vi "menu-SetWeights.vi"(10 "Start":i32, 11 "Array in":T1[](array[typedef])) -> (3 "Array out":T1[](array[typedef]))   [LabVIEW 2019]
uses:
  <resource>/Framework/Providers/API/mxLvMenuItem.ctl
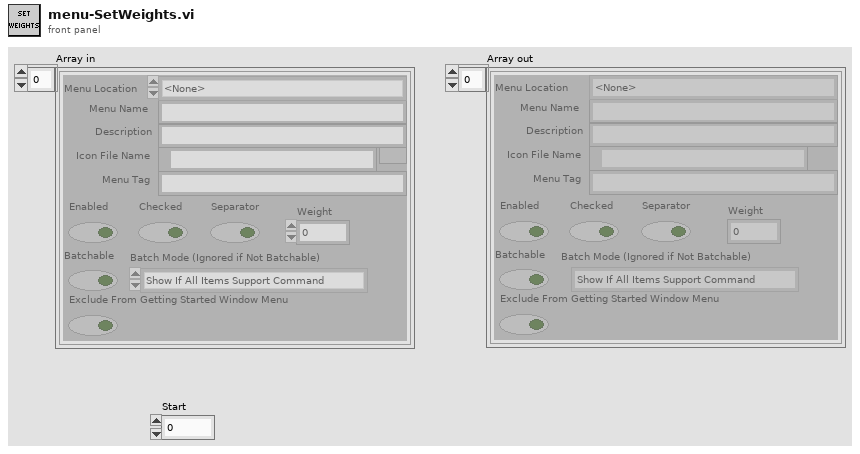
[diagram p1: front panel]
types:
  T1 = typedef "mxLvMenuItem.ctl" = cluster{"Menu Name":string, "Description":string, "Icon File Name":path, "Menu Tag":string, "Enabled":bool, "Checked":bool, "Separator":bool, "Batchable":bool, "Weight":i32, "Batch Mode (Ignored if Not Batchable)":enum32{"Show If All Items Support Command", "Show If Any Items Support Command"}, "Menu Location":enum32{"<None>", "Project", "Project / Build Specifications", "Tools", "Tools / Source Control", "Tools / Real-Time Module", "Help"}, "Exclude From Getting Started Window Menu":bool}
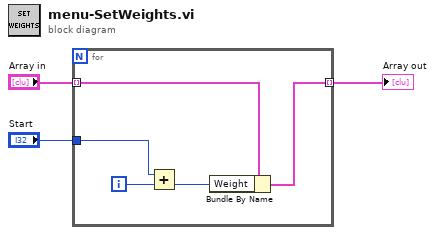
[diagram p0: block diagram]
diagram:
  n1 = for {
    tunnel: "Array in" -> [w8] mode=indexing
    tunnel: [w7] -> w2 mode=indexing
    tunnel: "Start" -> [w4]
    i -> [w6]
    n2 = Add(x=w4, y=w6) -> (x+y=w5:i32)
    n3 = Bundle By Name(cluster=w8, "Weight"=w5) -> (w7:T1)
  }
  "Array out" <- w2
